vi "Launcher_contador.vi"   [LabVIEW 2019]
uses:
  Contador_Bin_Actor.lvclass
  C:/Program Files/National Instruments/LabVIEW 2019/vi.lib/ActorFramework/Actor/Actor.lvclass
  <vilib>/ActorFramework/Actor/Actor.lvclass
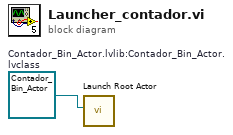
[diagram p0: block diagram]
diagram:
  w1 = refnum<class "Contador_Bin_Actor.lvclass"> refnum  # Contador_Bin_Actor.lvlib:Contador_Bin_Actor.lvclass
  n1 = call <vilib>:"Launch Root Actor.vi"("Actor"=w1) -> ()  [unwired: 9 in, 2 out]
